vi "Calculate push moves.vi"(7 "Position in":refnum<class "Position.lvclass">, 11 "Source":T1) -> (3 "Push moves":refnum<class "Move.lvclass">[](array[class]))   [LabVIEW 2016, in "Chesslib.lvlib" / "Pawn.lvclass"]
uses:
  Pawn.lvclass
  Position/Position.lvclass
  Moves/Move/Move.lvclass
  typedef/Square.ctl
  typedef/File.ctl
  typedef/Rank.ctl
  typedef/Neighbor.ctl
  Moves/Promotion/Promotion.lvclass
  C:/Users/GRTaggJ/Documents/Projects/chesslib/Moves/Move/Move.lvclass
  Moves/DoublePush/DoublePush.lvclass
  Chesslib.lvlib
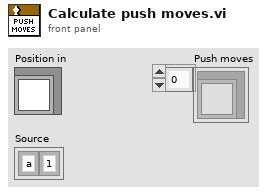
[diagram p1: front panel]
types:
  T1 = typedef "Chesslib.lvlib/Square.ctl" = cluster{"File":T2, "Rank":T3}
  T2 = typedef "Chesslib.lvlib/File.ctl" = enum8{"a", "b", "c", "d", "e", "f", "g", "h"}
  T3 = typedef "Chesslib.lvlib/Rank.ctl" = enum8{"1", "2", "3", "4", "5", "6", "7", "8"}
  T4 = typedef "Chesslib.lvlib/Color.ctl" = enum16{"Light", "Dark"}
  T5 = typedef "Chesslib.lvlib/Neighbor.ctl" = enum16{"N", "NW", "W", "SW", "S", "SE", "E", "NE", "vector"}
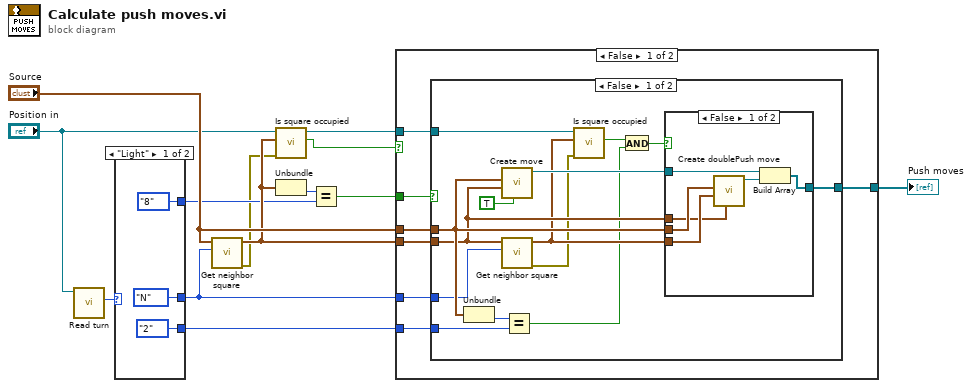
[diagram p0: block diagram]
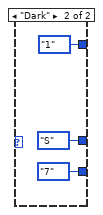
[diagram p2: hidden frame]
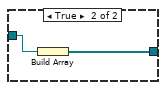
[diagram p3: hidden frame]
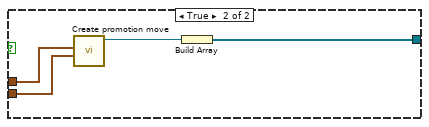
[diagram p4: hidden frame]
diagram:
  n1 = call "Read turn.vi"("Position in"="Position in") -> ("Turn"=w11:T4)  [unwired: 9 in, 1 out]
  n2 = case shown="\"Light\"" w11 {
    tunnel: [Neighbor."N" ("Neighbor (vector)") Neighbor."S" ("Neighbor (vector)")] -> w10
    tunnel: [Rank."2" ("Rank") Rank."7" ("Rank")] -> w7
    tunnel: [Rank."8" ("Rank") Rank."1" ("Rank")] -> w4
    frame "Light" {
    }
    frame "Dark" {
    }
  }
  n3 = call "Get neighbor square.vi"("Neighbor (vector)"=w10, "Square in"="Source") -> ("error out"=w2:errorcluster, "Square out"=w6:T1)  [unwired: 7 in, 1 out]
  n4 = call "Is square occupied.vi"("error in (no error)"=w2, "Square"=w6, "Position in"="Position in") -> ("Occupied"=w1:bool, "Position out"=w8:refnum<class "Position.lvclass">)  [unwired: 6 in, 1 out]
  n5 = Unbundle(w6) -> ("Rank"=w5:T3)  [unwired: 1 out]
  n6 = Equal?(x=w5, y=w4) -> (x = y?=w3:bool)
  n7 = case shown="False" w1 {
    tunnel: [w26 _] -> w13
    tunnel: "Source" -> [w25 _]
    tunnel: w10 -> [w24 _]
    tunnel: w8 -> [w23 _]
    tunnel: w7 -> [w22 _]
    tunnel: w6 -> [w21 _]
    tunnel: w3 -> [w20 _]
    frame False {
      n8 = case shown="False" w20 {
        tunnel: [w40 w49] -> w26
        tunnel: w25 -> [w39 w52]
        tunnel: w21 -> [w38 w51]
        tunnel: w24 -> [w37 _]
        tunnel: w23 -> [w36 _]
        tunnel: w22 -> [w35 _]
        frame False {
          n9 = Unbundle(w39) -> ("Rank"=w31:T3)  [unwired: 1 out]
          n10 = call "Create move.vi"("Pawn move (F)"=TRUE, "Destination"=w38, "Source"=w39) -> ("Move out"=w34:refnum<class "Move.lvclass">)  [unwired: 8 in]
          n11 = call "Get neighbor square.vi"("Neighbor (vector)"=w37, "Square in"=w38) -> ("error out"=w27:errorcluster, "Square out"=w33:T1)  [unwired: 7 in, 1 out]
          n12 = Equal?(x=w31, y=w35) -> (x = y?=w29:bool)
          n13 = call "Is square occupied.vi"("error in (no error)"=w27, "Square"=w33, "Position in"=w36) -> ("Occupied"=w28:bool)  [unwired: 6 in, 2 out]
          n14 = And(x=w28, y=w29) -> (x .and. y?=w30:bool)
          n15 = case shown="False" w30 {
            tunnel: w34 -> [w45 w48]
            tunnel: w39 -> [w42 _]
            tunnel: w33 -> [w46 _]
            tunnel: [w44 w47] -> w40
            tunnel: w38 -> [w41 _]
            frame False {
              n16 = call "Create doublePush move.vi"("enPassant target"=w41, "Destination"=w46, "Source"=w42) -> ("DoublePush move"=w43:refnum<class "DoublePush.lvclass">)  [unwired: 8 in]
              n17 = Build Array(w45, w43) -> (w44:refnum<class "Move.lvclass">[])
            }
            frame True {
              n18 = Build Array(w48) -> (w47:refnum<class "Move.lvclass">[])
            }
          }
        }
        frame True {
          n19 = call "Create promotion move.vi"("Destination"=w51, "Source"=w52) -> ("Promotion move"=w50:refnum<class "Promotion.lvclass">)  [unwired: 9 in]
          n20 = Build Array(w50) -> (w49:refnum<class "Promotion.lvclass">[])
        }
      }
    }
    frame True {
    }
  }
  "Push moves" <- w13
